vi "Pulse Width Modulation (FPGA, Use in SCTL).vi"(2 "PWM Period (Ticks)":u32=2000, 3 "PWM Duty Cycle (Ticks)":i32, 6 "Min Period (Ticks)":u32=1000, 7 "Sample Clock Advance (Ticks)":u32=9, 8 "Duty Limit (Ticks)":u32=100, 9 "PID Clock Advance (Ticks)":u32=50, 11 "Rate Limit (Ticks/Cycle)":i32=1000) -> (12 "Actual Duty Cycle (Ticks)":u32, 15 "PWM DO":bool, 16 "PID Clock":bool, 17 "Sample Clock":bool, 18 "Changed?":bool, 19 "Telapsed (Ticks)":u32)   [LabVIEW 2012]
doc: "Generates a digital pulse width modulation (PWM) signal. PWM signals are useful for driving loads such as motors and proportional valves because the average voltage supplied is equal to the PWM duty cycle. The output of this function can be connected to digital output modules. This function is designed for use in LabVIEW FPGA.\n\nOPERATION\nAt the beginning of each cycle the PWM Duty Cycle (Ticks) input is read and the PWM DO digital output is turned on. The digital output is left on for the amount of time specified by the PWM Duty Cycle (Ticks) input. The cycle repeats when the amount of time specified by the PWM Period (Ticks) has elapsed. The FPGA tick counter is used to calculate elapsed time. By default, one tick is equal to 25 nanoseconds (40 MHz), so a PWM Period (Ticks) of 2,000 results in a 20 kHz PWM signal. The PWM Duty Cycle (Ticks) input is a signed integer, but the sign of the value is ignored. Some applications use the sign of the PWM Duty Cycle (Ticks) signal to determine which direction to drive the motor.\n\nUse the rising edge of the PID Clock signal to trigger your FPGA-based current control PID loop execution. The rising edge of the PID Clock signal occurs just before the end of the PWM cycle. The amount of time before the end of the cycle the edge occurs is determined by the PID Clock Advance (Ticks) signal.\n\nUse the rising edge of the Sample Clock signal to trigger your analog input operation to read the motor current for closed loop control. The Sample Clock signal goes TRUE at the mid-point of the PWM DO output and goes FALSE at the beginning of the PWM cycle. For an inductive load, sampling the current at this time gives a rough estimate of the average current. The Sample Clock signal will continue to be generated even if the duty cycle is 0 or 100 percent. In those cases, the rising edge of the Sample Clock signal occurs at the beginning of the PWM cycle. The Sample Clock Advance (Ticks) signal is used to cause the rising edge to occur slightly before the PWM DO mid-point, to compensate for analog input sampling time. For the NI 9505 module, the analog input sampling occurs 9 FPGA clock ticks after the start of the FPGA I/O Node function.\n\nThe Telapsed (Ticks) signal can be used to trigger other operations at particular time in the PWM cycle. For instance, you could use this signal to trigger an analog input operation to occur once per PWM cycle at a programmable time within the PWM cycle. This counter resets back to 0 at the beginning of every PWM cycle.\n\nThe Min Period (Ticks) control is used to limit the PWM Period to prevent switching at frequencies that could damage the output MOSFETs in a digital output device. By default Min Period (Ticks) is set to 1000 ticks, which limits the PWM switching frequency to 40 kHz.\n\nThe Duty Limit (Ticks) control is used to limit the minimum ON and OFF time for the PWM output. If the Duty Cycle is less than the limit, it will be coerced to 0%. If the duty cycle is greater than the Period minus the Duty Limit, the Duty Cycle will be coerced to 100%. Some output devices such as the NI 9505 motor drive module require that the ON and OFF time not be less than a certain limit (2.5 microseconds for the NI 9505). By default Duty Limit (Ticks) is set to 100 ticks, or 2.5 microseconds.\n\nTo obtain the highest timing resolution when using this function in a loop, you can perform digital output I/O operations only when the PWM DO value has changed (rather than on every cycle). To do this, wire the Changed? output to the conditional terminal on a case structure and perform the I/O operation when the case is True. If the duty cycle is 0 or 100%, the Changed? output will strobe true once per PWM cycle at the beginning of the cycle.\n\nThis subVI is reentrant, so you can place multiple instances of the function in a LabVIEW FPGA application and they each will operate independently.\n\nINPUTS\nPWM Period (Ticks)- Total width of the pulse (inverse of the \"PWM Frequency\")\nPWM Duty Cycle (Ticks)- Time for which signal output stays True\nMin Period (Ticks)- The minimum allowed value for the PWM Period\nDuty Limit (Ticks)- The minimum allowed value for the PWM on time and off time\nPID Clock Advance (Ticks)- Determines how many clock ticks before the end of the PWM cycle that the PID Clock rising edge occurs\nSample Clock Advance (Ticks)- Determines how many clock ticks before the mid-point of the PWM digital output that the Sample Clock rising edge occurs \n\nOUTPUTS\nPWM DO- Digital PWM signal that can be connected to a digital output channel I/O node\nPID Clock- clock signal that can be used for synchronizing the execution of a current control PID loop\nSample Clock- clock signal that can be used to trigger an analog input operation to measure the average current in an inductive load\nChanged?- Value is True for one iteration when the PWM DO value has changed, or at the beginning of the PWM cycle if the duty cycle is 0 or 100%\nTelapsed- The amount of time elapsed during the current PWM cycle\n\nSCALING\n\nThe formulas below can be used for scaling from units of Hz, seconds, or percent duty cycle in the real-time host interface application. These formulas assume a 40 MHz (40,000,000 Ticks/sec) FPGA clock rate.\n\nPWM Period (Ticks) = 40,000,000 / PWM Period (Hz)\nPWM Period (Ticks) = 40,000,000 * PWM Period (sec)\nPWM Duty Cycle (Ticks) = PWM Period (Ticks) * PWM Duty Cycle (%) / 100\nPWM Duty Cycle (Ticks) = 40,000,000 * PWM Duty Cycle (sec)"
uses:
  Instance           1 50Saved   Pulse Width Modulation (FPGA, Use in SCTL) .vi
  Instance           2 50Saved   Pulse Width Modulation (FPGA, Use in SCTL) .vi
  <vilib>/rvi/Arithmetic/AddSubMult/XNode/nirviSatArithmetic.xnode
panel:
  out "R4 (Rate Lim. Duty)":i32
  out "R4 (Latched Period)":u32
  out "R3 (Ton)":u32
  out "R2 (Reset)":bool
  out "R1 (Latched Duty Cycle)":i32
  # "Internal Registers"
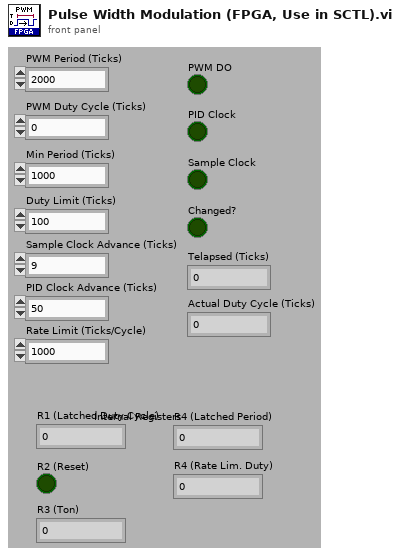
[diagram p1: front panel]
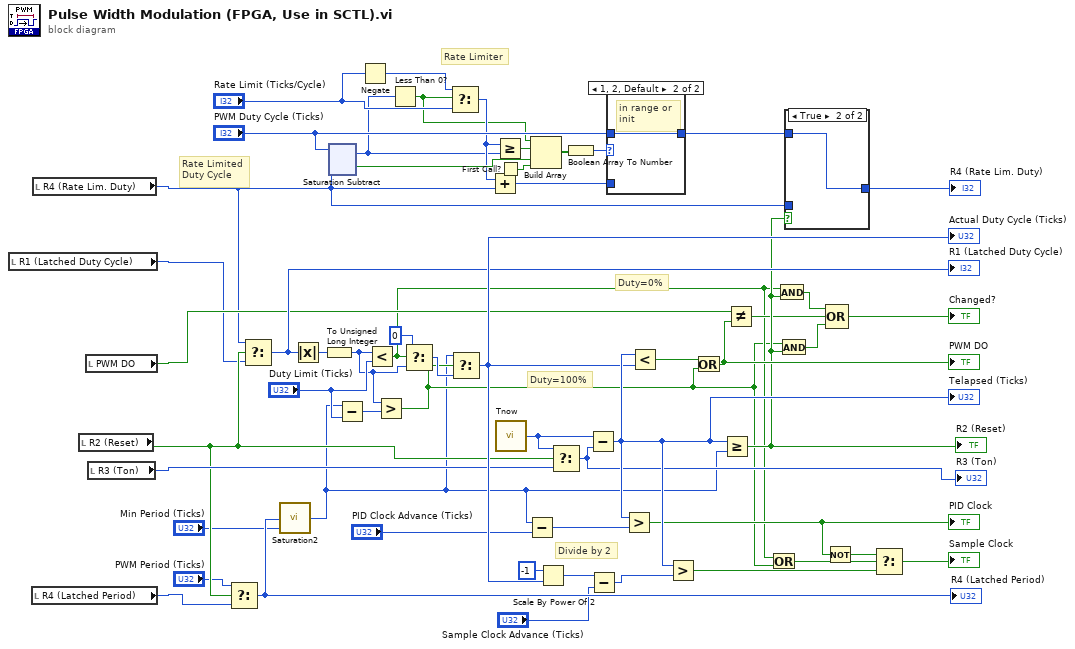
[diagram p0: block diagram]
diagram:
  # "Rate Limiter"
  # "Rate Limited\nDuty Cycle"
  # "Duty=100%"
  # "Duty=0%"
  # "Divide by 2"
  n1 = local read "R1 (Latched Duty Cycle)"() -> (w40:i32)
  n2 = local read "R4 (Latched Period)"() -> (w44:u32)
  n3 = local read "R4 (Rate Lim. Duty)"() -> (w39:i32)
  n4 = local read "R2 (Reset)"() -> (w42:bool)
  n5 = local read "PWM DO"() -> (w41:bool)
  n6 = local read "R3 (Ton)"() -> (w43:u32)
  n7 = Select(t="PWM Period (Ticks)", s=w42, f=w44) -> (s? t:f=w47:u32)
  "R4 (Latched Period)" <- w47
  n8 = Select(t=w39, s=w42, f=w40) -> (s? t:f=w49:i32)
  "R1 (Latched Duty Cycle)" <- w49
  n9 = call "Saturation2"("input"=w47, "lower limit"="Min Period (Ticks)") -> ("output"=w14:u32)  [unwired: 7 in]
  n10 = Absolute Value(x=w49) -> (abs(x)=w34:i32)
  n11 = To Unsigned Long Integer(number=w34) -> (unsigned 32bit integer=w29:u32)
  n12 = xnode ("Saturation Subtract")("x"="PWM Duty Cycle (Ticks)", "y"=w39) -> ("x-y"=w1:i32, "overflow"=w10:bool)
  n13 = Subtract(x=w14, y="Duty Limit (Ticks)") -> (x-y=w27:u32)
  n14 = Negate(x="Rate Limit (Ticks/Cycle)") -> (-x=w11:i32)
  n15 = Less?(x=w29, y="Duty Limit (Ticks)") -> (x < y?=w25:bool)
  n16 = Greater?(x=w29, y=w27) -> (0:w24:bool)
  n17 = Less Than 0?(x=w1) -> (x < 0?=w2:bool)
  n18 = Select(t=u32 0, s=w25, f=w29) -> (s? t:f=w28:u32)
  n19 = Select(t=w11, s=w2, f="Rate Limit (Ticks/Cycle)") -> (s? t:f=w8:i32)
  n20 = Select(t=w14, s=w24, f=w28) -> (s? t:f=w50:u32)
  "Actual Duty Cycle (Ticks)" <- w50
  n21 = Add(x=w8, y=w39) -> (x+y=w9:i32)
  n22 = Greater Or Equal?(x=w8, y=w1) -> (x >= y?=w5:bool)
  n23 = First Call?() -> (First Call?: T/F=w3:bool)
  n24 = call "Tnow"() -> ("Tick Count(Ticks)"=w38:u32)
  n25 = Subtract(x=w14, y="PID Clock Advance (Ticks)") -> (x-y=w16:u32)
  n26 = Build Array(w2, w5, w10, w3) -> (w6:bool[])
  n27 = Scale By Power Of 2(n=i8 -1, x=w50) -> (x*2^n=w19:u32)
  n28 = Select(t=w38, s=w42, f=w43) -> (s? t:f=w48:u32)
  "R3 (Ton)" <- w48
  n29 = Boolean Array To Number(Boolean array=w6) -> (number=w7:u8)
  n30 = Subtract(x=w38, y=w48) -> (x-y=w55:u32)
  "Telapsed (Ticks)" <- w55
  n31 = Subtract(x=w19, y="Sample Clock Advance (Ticks)") -> (x-y=w18:u32)
  n32 = case shown="1, 2, Default" w7 {
    tunnel: w9 -> [w56 _]
    tunnel: "PWM Duty Cycle (Ticks)" -> [_ w57]
    tunnel: [w56 w57] -> w4
    frame 0, 3..7 {
      # "out of range"
    }
    frame 1, 2, Default {
      # "in range or \ninit"
    }
  }
  n33 = Greater?(x=w55, y=w16) -> (0:w54:bool)
  "PID Clock" <- w54
  n34 = Less?(x=w55, y=w50) -> (x < y?=w36:bool)
  n35 = Greater?(x=w55, y=w18) -> (0:w21:bool)
  n36 = Or(x=w36, y=w24) -> (x .or. y?=w53:bool)
  "PWM DO" <- w53
  n37 = Greater Or Equal?(x=w55, y=w14) -> (x >= y?=w45:bool)
  "R2 (Reset)" <- w45
  n38 = Not Equal?(x=w41, y=w53) -> (x != y?=w37:bool)
  n39 = Or(x=w25, y=w24) -> (x .or. y?=w23:bool)
  n40 = And(x=w25, y=w45) -> (x .and. y?=w33:bool)
  n41 = And(x=w24, y=w45) -> (x .and. y?=w32:bool)
  n42 = case shown="True" w45 {
    tunnel: [w58 w59] -> w46
    tunnel: w4 -> [_ w59]
    tunnel: w39 -> [w58 _]
    frame False {
    }
    frame True {
    }
  }
  "R4 (Rate Lim. Duty)" <- w46
  n43 = Not(x=w54) -> (.not. x?=w22:bool)
  n44 = Compound Arithmetic op=OR(w33, w37, w32) -> (→"Changed?":bool)
  n45 = Select(t=w22, s=w23, f=w21) -> (s? t:f=→"Sample Clock":bool)
